vi "Send Response Without Parameters.vi"(8 "error in (no error)":errorcluster, 9 "timeout in ms (0)":i32 format="%d ms", 10 "response":T1, 11 "Plugin Thread in":refnum<class "Plugin Thread.lvclass">) -> (0 "error out":errorcluster, 3 "Plugin Thread out":refnum<class "Plugin Thread.lvclass">)   [LabVIEW 2017, in "DSF Core.lvlib" / "Plugin Thread.lvclass"]
uses:
  Thread/Plugin/Plugin Thread.lvclass
  Interface/Plugin/Response.ctl
  Interface/Plugin/Response Data.ctl
  Interface/Plugin/Response Parameters.ctl
  Interface/Plugin/Send Plugin Response.vi
  Interface/Plugin/Plugin Interface.lvclass
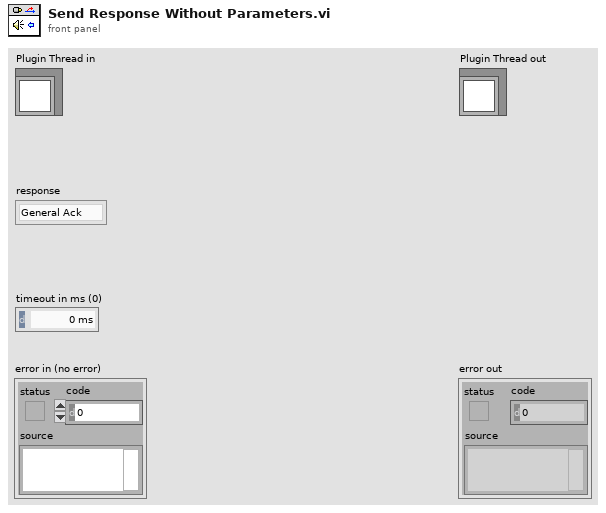
[diagram p1: front panel]
types:
  T1 = typedef "DSF Core.lvlib/Plugin Interface.lvclass/Response.ctl" = enum8{"General Ack", "Shutting Down"}
  T2 = typedef "DSF Core.lvlib/Plugin Interface.lvclass/Response Data.ctl" = cluster{"Response":T1, "Parameters":T3}
  T3 = typedef "DSF Core.lvlib/Plugin Interface.lvclass/Response Parameters.ctl" = cluster{"arg1":u64, "arg2":u64}
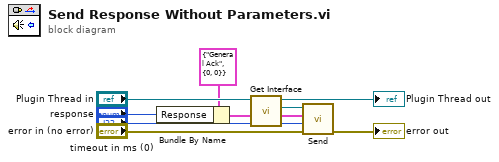
[diagram p0: block diagram]
diagram:
  n1 = Bundle By Name(cluster=T2 {"Response"=enum."General Ack", "Parameters"={"arg1"=0, "arg2"=0}} ("response"), "Response"="response") -> (w2:T2)
  n2 = call "Get Interface.vi"("Transceiver Thread in"="Plugin Thread in") -> ("Interface"=w8:refnum<class "Plugin Interface.lvclass">, "Transceiver Thread out"=→"Plugin Thread out":refnum<class "Plugin Thread.lvclass">)  [unwired: 9 in]
  n3 = call-poly "Send.vi"("error in (no error)"="error in (no error)", "timeout in ms (0)"="timeout in ms (0)", "response"=w2, "Plugin Interface in"=w8) -> ("error out"=→"error out":errorcluster)  [unwired: 6 in, 1 out]
